vi "WriteHeaderTwoHands.vi"(8 "Error in":errorcluster) -> (0 "Error out":errorcluster, 2 "Header string array":string[](array[string]))   [LabVIEW 2017, in "LeapMotion.lvlib"]
uses:
  LeapMotion.lvlib
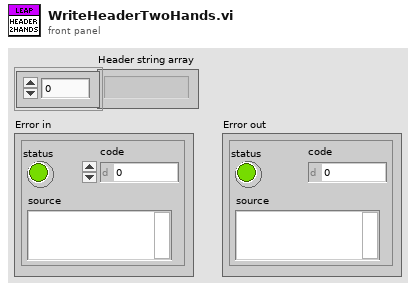
[diagram p1: front panel]
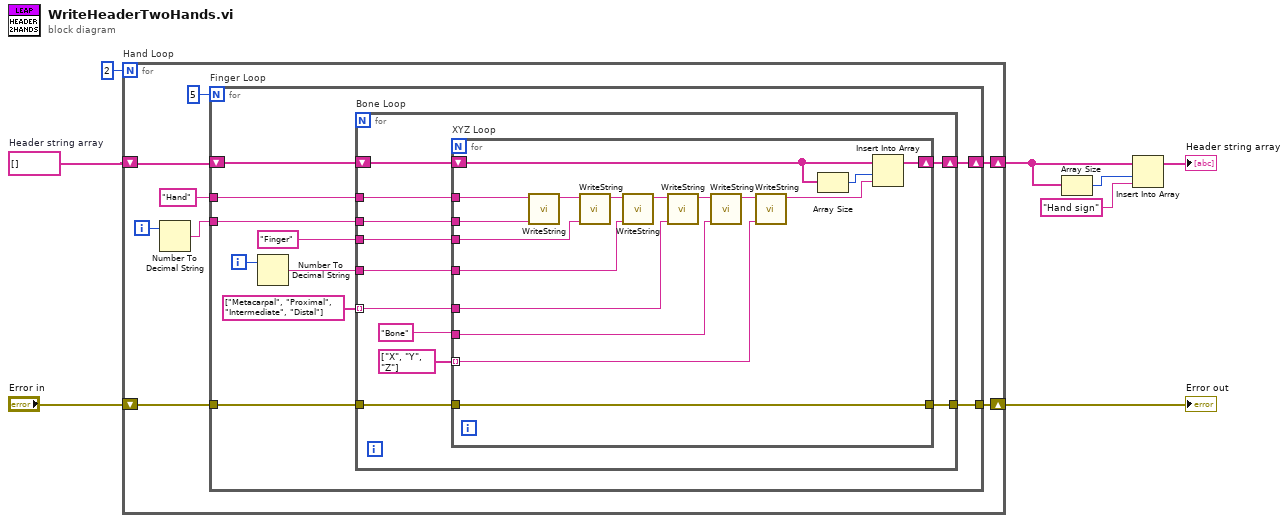
[diagram p0: block diagram]
diagram:
  w2 = string[] []  # Header string array
  n1 = for "Hand Loop" {
    N: 2 -> [_]
    shift-right: [w9] -> w4
    shift-left: "Error in" -> [w10]
    shift-right: [w16] -> w7
    shift-left: w2 -> [w14]
    i -> [w13]
    n2 = Number To Decimal String(number=w13) -> (decimal integer string=w12:string)  [unwired: 1 in]
    n3 = for "Finger Loop" {
      N: 5 -> [_]
      shift-right: [w26] -> w16
      shift-left: w14 -> [w23]
      tunnel: w12 -> [w20]
      tunnel: "Hand" -> [w19]
      tunnel: w10 -> [w18]
      tunnel: [w17] -> w9
      i -> [w25]
      n4 = Number To Decimal String(number=w25) -> (decimal integer string=w21:string)  [unwired: 1 in]
      n5 = for "Bone Loop" {
        tunnel: string[] ["Metacarpal", "Proximal", "Intermediate", "Distal"] ("Bone name") -> [w35] mode=indexing
        shift-right: [w36] -> w26
        shift-left: w23 -> [w37]
        tunnel: "Finger" -> [w34]
        tunnel: w21 -> [w33]
        tunnel: w20 -> [w32]
        tunnel: w19 -> [w31]
        tunnel: w18 -> [w28]
        tunnel: [w27] -> w17
        n6 = for "XYZ Loop" {
          tunnel: string[] ["X", "Y", "Z"] ("Dimension") -> [w39] mode=indexing
          shift-right: [w54] -> w36
          shift-left: w37 -> [w53]
          tunnel: w35 -> [w50]
          tunnel: "Bone" -> [w48]
          tunnel: w34 -> [w41]
          tunnel: w33 -> [w46]
          tunnel: w31 -> [w44]
          tunnel: w32 -> [w43]
          tunnel: w28 -> [w38]
          tunnel: [w38] -> w27
          n7 = call "WriteString.vi"("To apppend"=w43, "Original string"=w44) -> ("Appended string"=w42:string)  [unwired: 9 in]
          n8 = call "WriteString.vi"("To apppend"=w41, "Original string"=w42) -> ("Appended string"=w40:string)  [unwired: 9 in]
          n9 = call "WriteString.vi"("To apppend"=w46, "Original string"=w40) -> ("Appended string"=w51:string)  [unwired: 9 in]
          n10 = call "WriteString.vi"("To apppend"=w50, "Original string"=w51) -> ("Appended string"=w49:string)  [unwired: 9 in]
          n11 = call "WriteString.vi"("To apppend"=w48, "Original string"=w49) -> ("Appended string"=w47:string)  [unwired: 9 in]
          n12 = call "WriteString.vi"("To apppend"=w39, "Original string"=w47) -> ("Appended string"=w45:string)  [unwired: 9 in]
          n13 = Array Size(array=w53) -> (size(s)=w52:i32)
          n14 = Insert Into Array(array=w53, index=w52, new element=w45) -> (w54:string[])
        }
      }
    }
  }
  "Error out" <- w4
  n15 = Array Size(array=w7) -> (size(s)=w6:i32)
  n16 = Insert Into Array(array=w7, index=w6, new element="Hand sign") -> (→"Header string array":string[])
